vi "SubVI_ReadTitle.vi"(11 "String":string) -> (3 "Title":string[](array[string]))   [LabVIEW 2011]
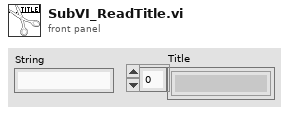
[diagram p1: front panel]
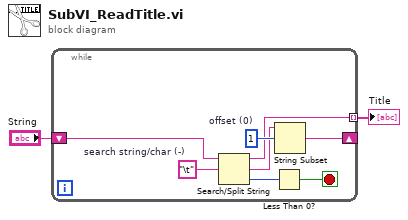
[diagram p0: block diagram]
diagram:
  n1 = while {
    shift-right: [w6] -> _
    shift-left: "String" -> [w10]
    tunnel: [w3] -> w1 mode=indexing
    stop <- w5 stop-if-true
    w8 = 1  # offset (0)
    w9 = "\t"  # search string/char (-)
    n2 = Search/Split String(string=w10, search string/char (-)=w9) -> (substring before match=w3:string, match + rest of string=w7:string, offset of match=w4:i32)  [unwired: 1 in]
    n3 = Less Than 0?(x=w4) -> (x < 0?=w5:bool)
    n4 = String Subset(string=w7, offset (0)=w8) -> (substring=w6:string)  [unwired: 1 in]
  }
  "Title" <- w1
